vi "Get Error Details (Error 1172).vi"(11 "error":errorcluster) -> (1 "Message":string, 2 "Stack Trace":string, 3 "Type":string)   [LabVIEW 2013, in "JUnit Conversion.lvlib"]
uses:
  JUnit Conversion.lvlib
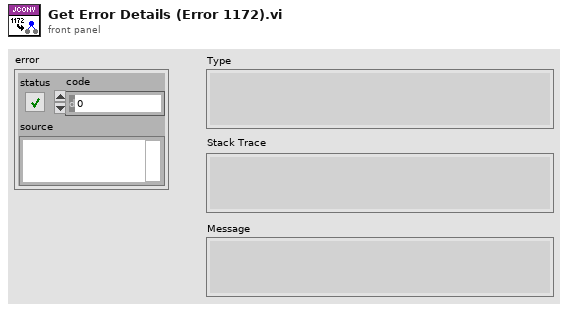
[diagram p1: front panel]
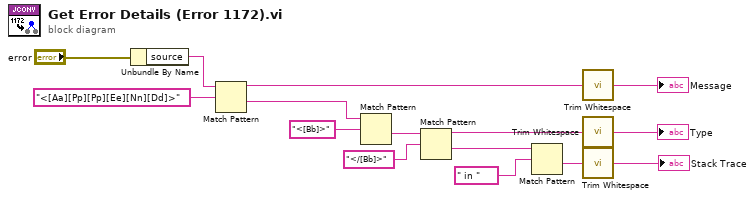
[diagram p0: block diagram]
diagram:
  n1 = Unbundle By Name("error") -> ("source"=w1:string)
  n2 = Match Pattern(string=w1, regular expression="<[Aa][Pp][Pp][Ee][Nn][Dd]>") -> (before substring=w13:string, after substring=w9:string)  [unwired: 1 in, 2 out]
  n3 = Match Pattern(string=w9, regular expression="<[Bb]>") -> (after substring=w12:string)  [unwired: 1 in, 3 out]
  n4 = Match Pattern(string=w12, regular expression="</[Bb]>") -> (before substring=w8:string, after substring=w7:string)  [unwired: 1 in, 2 out]
  n5 = Match Pattern(string=w7, regular expression=" in ") -> (after substring=w5:string)  [unwired: 1 in, 3 out]
  n6 = call <vilib>:"Trim Whitespace.vi"("string"=w13) -> ("trimmed string"=→"Message":string)  [unwired: 1 in]
  n7 = call <vilib>:"Trim Whitespace.vi"("string"=w8) -> ("trimmed string"=→"Type":string)  [unwired: 1 in]
  n8 = call <vilib>:"Trim Whitespace.vi"("string"=w5) -> ("trimmed string"=→"Stack Trace":string)  [unwired: 1 in]
